vi "Set Columns Count.vi"(8 "error in":errorcluster, 10 "ColumnsCount":i32, 11 "SourceGrid in":refnum<class "SourceGrid.lvclass">) -> (0 "error out":errorcluster, 3 "SourceGrid out":refnum<class "SourceGrid.lvclass">)   [LabVIEW 2023, in "SourceGrid.lvlib" / "SourceGrid.lvclass"]
uses:
  SourceGrid.lvclass
  SourceGrid.lvclass/SourceGrid.ctl
  D:/git/Sourcegrid-LabVIEW/dll/SourceGrid.dll
  dll/SourceGrid.dll
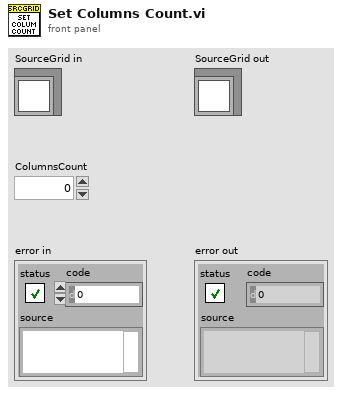
[diagram p1: front panel]
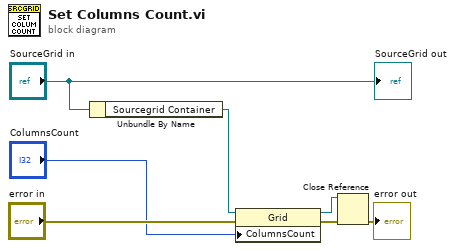
[diagram p0: block diagram]
diagram:
  n1 = Unbundle By Name("SourceGrid in") -> ("Sourcegrid Container"=w6:refnum<k24>)
  n2 = property class="Grid"(reference=w6, error in="error in", "ColumnsCount"="ColumnsCount") -> (reference out=w1:refnum<k24>, error out=w4:errorcluster)
  n3 = Close Reference(reference=w1, error in (no error)=w4) -> (error out=→"error out":errorcluster)
  "SourceGrid out" <- "SourceGrid in"
